vi "subGetAssemblyHintPaths.vi"(0 "VeriStand assembly version string (2014.0.0.0)":string, 5 "VeriStand GAC assembly version (4.0.2014.0.0.0)":string, 7 "TestStand version string (2014)":string, 9 "TestStand assembly version (2014.0.0.0)":string, 11 "error in":errorcluster) -> (4 "New Assembly Hint Paths":string[](array[string]), 6 "New Assembly Include Paths":string[](array[string]), 15 "error out":errorcluster)   [LabVIEW 2015, in "veristand-steps-build-tools.lvlib"]
uses:
  veristand-steps-build-tools.lvlib
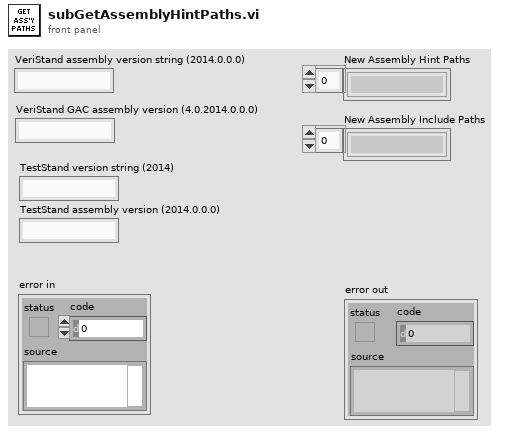
[diagram p1: front panel]
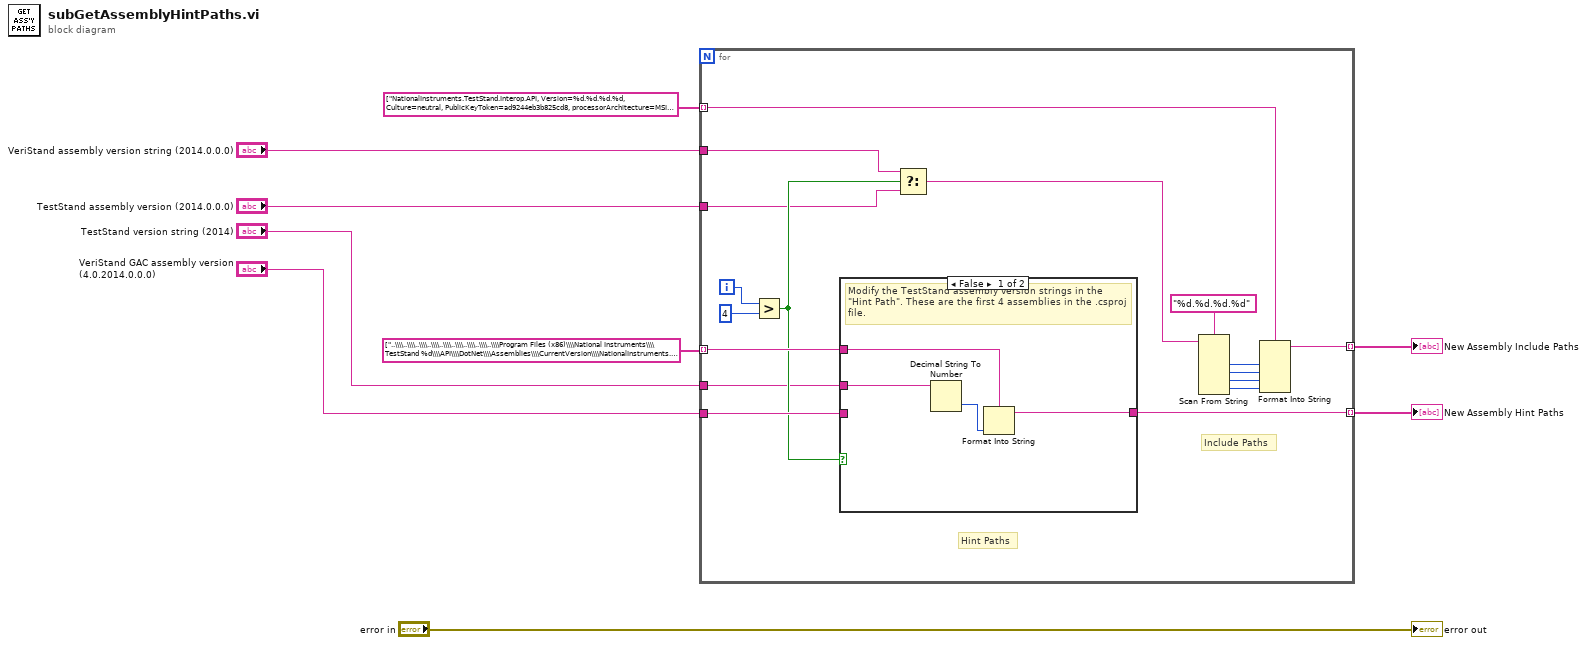
[diagram p0: block diagram]
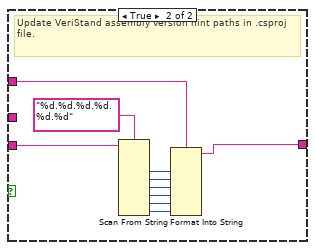
[diagram p2: hidden frame]
diagram:
  n1 = for {
    tunnel: [w22] -> w7 mode=indexing
    tunnel: string[] ["..\\\\..\\\\..\\\\..\\\\..\\\\..\\\\..\\\\..\\\\..\\\\Program Files (x86)\\\\National Instruments\\\\TestStand %d\\\\API\\\\DotNet\\\\Assemblies\\\\CurrentVersion\\\\NationalInstruments.TestStand.Interop.API.dll", "..\\\\..\\\\..\\\\..\\\\..\\\\..\\\\..\\\\..\\\\..\\\\Program Files (x86)\\\\National Instruments\\\\TestStand %d\\\\API\\\\DotNet\\\\Assemblies\\\\CurrentVersion\\\\NationalInstruments.TestStand.Interop.UI.dll", "..\\\\..\\\\..\\\\..\\\\..\\\\..\\\\..\\\\..\\\\..\\\\Program Files (x86)\\\\National Instruments\\\\TestStand %d\\\\API\\\\DotNet\\\\Assemblies\\\\CurrentVersion\\\\NationalInstruments.TestStand.Interop.UI.AxControls.dll", "..\\\\..\\\\..\\\\..\\\\..\\\\..\\\\..\\\\..\\\\..\\\\Program Files (x86)\\\\National Instruments\\\\TestStand %d\\\\API\\\\DotNet\\\\Assemblies\\\\CurrentVersion\\\\NationalInstruments.TestStand.Interop.UISupport.dll", "..\\\\..\\\\..\\\\..\\\\..\\\\..\\\\..\\\\..\\\\..\\\\Program Files (x86)\\\\National Instruments\\\\TestStand %d\\\\Bin\\\\NationalInstruments.TestStand.Utility.dll", "..\\\\..\\\\..\\\\..\\\\..\\\\..\\\\..\\\\..\\\\Windows\\\\Microsoft.NET\\\\assembly\\\\GAC_MSIL\\\\NationalInstruments.VeriStand\\\\v%d.%d_%d.%d.%d.%d__a6d690c380daa308\\\\NationalInstruments.VeriStand.dll", "..\\\\..\\\\..\\\\..\\\\..\\\\..\\\\..\\\\..\\\\Windows\\\\Microsoft.NET\\\\assembly\\\\GAC_MSIL\\\\NationalInstruments.VeriStand.ClientAPI\\\\v%d.%d_%d.%d.%d.%d__a6d690c380daa308\\\\NationalInstruments.VeriStand.ClientAPI.dll", "..\\\\..\\\\..\\\\..\\\\..\\\\..\\\\..\\\\..\\\\Windows\\\\Microsoft.NET\\\\assembly\\\\GAC_MSIL\\\\NationalInstruments.VeriStand.DataTypes\\\\v%d.%d_%d.%d.%d.%d__a6d690c380daa308\\\\NationalInstruments.VeriStand.DataTypes.dll", "..\\\\..\\\\..\\\\..\\\\..\\\\..\\\\..\\\\..\\\\Windows\\\\Microsoft.NET\\\\assembly\\\\GAC_MSIL\\\\NationalInstruments.VeriStand.RealTimeSequenceDefinitionAPI\\\\v%d.%d_%d.%d.%d.%d__a6d690c380daa308\\\\NationalInstruments.VeriStand.RealTimeSequenceDefinitionAPI.dll", "..\\\\..\\\\..\\\\..\\\\..\\\\..\\\\..\\\\..\\\\Windows\\\\Microsoft.NET\\\\assembly\\\\GAC_MSIL\\\\NationalInstruments.VeriStand.SystemDefinitionAPI\\\\v%d.%d_%d.%d.%d.%d__a6d690c380daa308\\\\NationalInstruments.VeriStand.SystemDefinitionAPI.dll", "..\\\\..\\\\..\\\\..\\\\..\\\\..\\\\..\\\\..\\\\Windows\\\\Microsoft.NET\\\\assembly\\\\GAC_MSIL\\\\NationalInstruments.VeriStand.SystemStorage\\\\v%d.%d_%d.%d.%d.%d__a6d690c380daa308\\\\NationalInstruments.VeriStand.SystemStorage.dll", "..\\\\..\\\\..\\\\..\\\\..\\\\..\\\\..\\\\..\\\\Windows\\\\Microsoft.NET\\\\assembly\\\\GAC_MSIL\\\\NationalInstruments.VeriStand.SystemStorageUI\\\\v%d.%d_%d.%d.%d.%d__a6d690c380daa308\\\\NationalInstruments.VeriStand.SystemStorageUI.dll", "..\\\\..\\\\..\\\\..\\\\..\\\\..\\\\..\\\\..\\\\Windows\\\\Microsoft.NET\\\\assembly\\\\GAC_MSIL\\\\NationalInstruments.VeriStand.WorkspaceMacro\\\\v%d.%d_%d.%d.%d.%d__a6d690c380daa308\\\\NationalInstruments.VeriStand.WorkspaceMacro.dll"] -> [w21] mode=indexing
    tunnel: [w20] -> w8 mode=indexing
    tunnel: "VeriStand GAC assembly version (4.0.2014.0.0.0)" -> [w18]
    tunnel: "VeriStand assembly version string (2014.0.0.0)" -> [w16]
    tunnel: "TestStand version string (2014)" -> [w11]
    tunnel: string[] ["NationalInstruments.TestStand.Interop.API, Version=%d.%d.%d.%d, Culture=neutral, PublicKeyToken=ad9244eb3b825cd8, processorArchitecture=MSIL", "NationalInstruments.TestStand.Interop.UI, Version=%d.%d.%d.%d, Culture=neutral, PublicKeyToken=ad9244eb3b825cd8, processorArchitecture=MSIL", "NationalInstruments.TestStand.Interop.UI.AxControls, Version=%d.%d.%d.%d, Culture=neutral, PublicKeyToken=ad9244eb3b825cd8, processorArchitecture=MSIL", "NationalInstruments.TestStand.Interop.UI.Support, Version=%d.%d.%d.%d, Culture=neutral, PublicKeyToken=ad9244eb3b825cd8, processorArchitecture=MSIL", "NationalInstruments.TestStand.Interop.Utility, Version=%d.%d.%d.%d, Culture=neutral, processorArchitecture=x86", "NationalInstruments.VeriStand, Version=%d.%d.%d.%d, Culture=neutral, PublicKeyToken=a6d690c380daa308, processorArchitecture=MSIL", "NationalInstruments.VeriStand.ClientAPI, Version=%d.%d.%d.%d, Culture=neutral, PublicKeyToken=a6d690c380daa308, processorArchitecture=MSIL", "NationalInstruments.VeriStand.DataTypes, Version=%d.%d.%d.%d, Culture=neutral, PublicKeyToken=a6d690c380daa308, processorArchitecture=MSIL", "NationalInstruments.VeriStand.RealTimeSequenceDefinitionApi, Version=%d.%d.%d.%d, Culture=neutral, PublicKeyToken=a6d690c380daa308, processorArchitecture=MSIL", "NationalInstruments.VeriStand.SystemDefinitionAPI, Version=%d.%d.%d.%d, Culture=neutral, PublicKeyToken=a6d690c380daa308, processorArchitecture=MSIL", "NationalInstruments.VeriStand.SystemStorage, Version=%d.%d.%d.%d, Culture=neutral, PublicKeyToken=a6d690c380daa308, processorArchitecture=MSIL", "NationalInstruments.VeriStand.SystemStorageUI, Version=%d.%d.%d.%d, Culture=neutral, PublicKeyToken=a6d690c380daa308, processorArchitecture=MSIL", "NationalInstruments.VeriStand.WorkspaceMacro, Version=%d.%d.%d.%d, Culture=neutral, PublicKeyToken=a6d690c380daa308, processorArchitecture=MSIL"] -> [w13] mode=indexing
    tunnel: "TestStand assembly version (2014.0.0.0)" -> [w10]
    i -> [w19]
    # "Hint Paths"
    # "Include Paths"
    n2 = Greater?(x=w19, y=4 ("x")) -> (0:w17:bool)
    n3 = case shown="False" w17 {
      tunnel: w21 -> [w30 w40]
      tunnel: [w29 w39] -> w20
      tunnel: w18 -> [_ w38]
      tunnel: w11 -> [w27 _]
      frame False {
        # "Modify the TestStand assembly version strings in the \"Hint Path\". These are the first 4 assemblies in the .csproj file."
        n4 = Decimal String To Number(string=w27) -> (number=w28:i32)  [unwired: 2 in, 1 out]
        n5 = Format Into String(format string=w30, w28) -> (resulting string=w29:string)  [unwired: 2 in, 1 out]
      }
      frame True {
        # "Update VeriStand assembly version hint paths in .csproj file."
        n6 = Scan From String(format string="%d.%d.%d.%d.%d.%d", input string=w38) -> (output 1=w37:i32, output 2=w36:i32, output 3=w35:i32, output 4=w34:i32, output 5=w33:i32, output 6=w32:i32)  [unwired: 8 in, 3 out]
        n7 = Format Into String(format string=w40, w37, w36, w35, w34, w33, w32) -> (resulting string=w39:string)  [unwired: 2 in, 1 out]
      }
    }
    n8 = Select(t=w16, s=w17, f=w10) -> (s? t:f=w15:string)
    n9 = Scan From String(format string="%d.%d.%d.%d", input string=w15) -> (output 1=w26:i32, output 2=w25:i32, output 3=w24:i32, output 4=w23:i32)  [unwired: 6 in, 3 out]
    n10 = Format Into String(format string=w13, w26, w25, w24, w23) -> (resulting string=w22:string)  [unwired: 2 in, 1 out]
  }
  "New Assembly Include Paths" <- w7
  "New Assembly Hint Paths" <- w8
  "error out" <- "error in"
